vi "WriteToLogFile.vi"(8 "error in":errorcluster, 10 "File content in":string, 11 "MassCompile in":refnum<class "MassCompile.lvclass">) -> (0 "error out":errorcluster, 2 "File content out":string, 3 "MassCompile out":refnum<class "MassCompile.lvclass">)   [LabVIEW 2014, in "MassCompile.lvclass"]
uses:
  MassCompile.lvclass
  MassCompile.lvclass/MassCompile.ctl
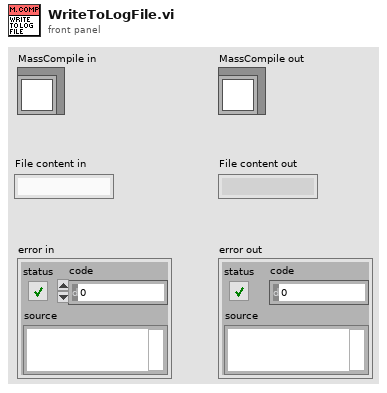
[diagram p1: front panel]
types:
  T1 = enum16{"open", "replace", "create", "open or create", "replace or create", "replace or create with confirmation"}
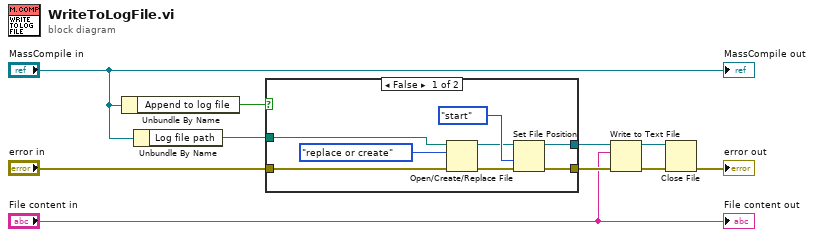
[diagram p0: block diagram]
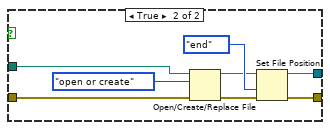
[diagram p2: hidden frame]
diagram:
  n1 = Unbundle By Name("MassCompile in") -> ("Append to log file"=w8:bool)
  n2 = Unbundle By Name("MassCompile in") -> ("Log file path"=w5:path)
  n3 = case shown="False" w8 {
    tunnel: [w18 w25] -> w9
    tunnel: [w17 w24] -> w10
    tunnel: "error in" -> [w14 w20]
    tunnel: w5 -> [w11 w19]
    frame False {
      n4 = Open/Create/Replace File(file path (use dialog)=w11, error in=w14, operation (0:open)=T1."replace or create") -> (refnum out=w15:refnum<file>, error out=w13:errorcluster)  [unwired: 3 in, 1 out]
      n5 = Set File Position(refnum=w15, from (0:start)=enum16{"start", "end", "current"}."start", error in=w13) -> (refnum out=w18:refnum<file>, error out=w17:errorcluster)  [unwired: 1 in]
    }
    frame True {
      n6 = Open/Create/Replace File(file path (use dialog)=w19, error in=w20, operation (0:open)=T1."open or create") -> (refnum out=w22:refnum<file>, error out=w21:errorcluster)  [unwired: 3 in, 1 out]
      n7 = Set File Position(refnum=w22, from (0:start)=enum16{"start", "end", "current"}."end", error in=w21) -> (refnum out=w25:refnum<file>, error out=w24:errorcluster)  [unwired: 1 in]
    }
  }
  n8 = Write to Text File(file (use dialog)=w9, text="File content in", error in=w10) -> (refnum out=w1:refnum<file>, error out=w3:errorcluster)  [unwired: 1 in, 1 out]
  n9 = Close File(refnum=w1, error in=w3) -> (error out=→"error out":errorcluster)  [unwired: 1 out]
  "MassCompile out" <- "MassCompile in"
  "File content out" <- "File content in"
